vi "Asynchronous Write.vi"(8 "error in":errorcluster, 10 "Data In":string, 11 "Serial Session in":refnum<class "Serial Session.lvclass">) -> (0 "error out":errorcluster, 3 "Serial Session out":refnum<class "Serial Session.lvclass">)   [LabVIEW 2016, in "Serial Session.lvclass"]
doc: "Asynchronous write to port."
uses:
  Serial Session.lvclass
  Serial Session.lvclass/Serial Session.ctl
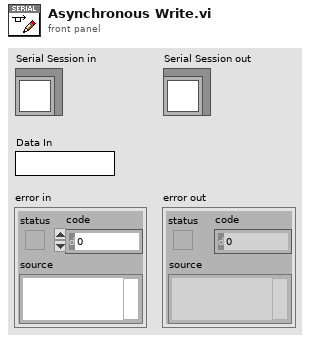
[diagram p1: front panel]
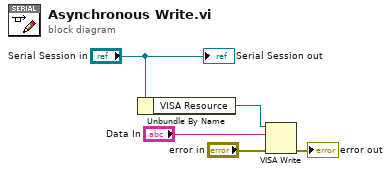
[diagram p0: block diagram]
diagram:
  n1 = Unbundle By Name("Serial Session in") -> ("VISA Resource"=w4:refnum<visa-resource-name>)
  n2 = VISA Write(VISA resource name=w4, write buffer="Data In", error in (no error)="error in") -> (error out=→"error out":errorcluster)  [unwired: 2 out]
  "Serial Session out" <- "Serial Session in"
